vi "All stations power supply ID config.vi"(10 "station idx":i32, 11 "configuration file path":path) -> (0 "error out":errorcluster caption="错误输出", 2 "station idx":i32, 3 "configuration file path":path, 5 "one state power supply":T1={"VISA name CH"="", "Voltage Level (12 V)"=14.0, "Current Level (30 A)"=30.0})   [LabVIEW 2018]
uses:
  Crl defs/one state power supply config.ctl
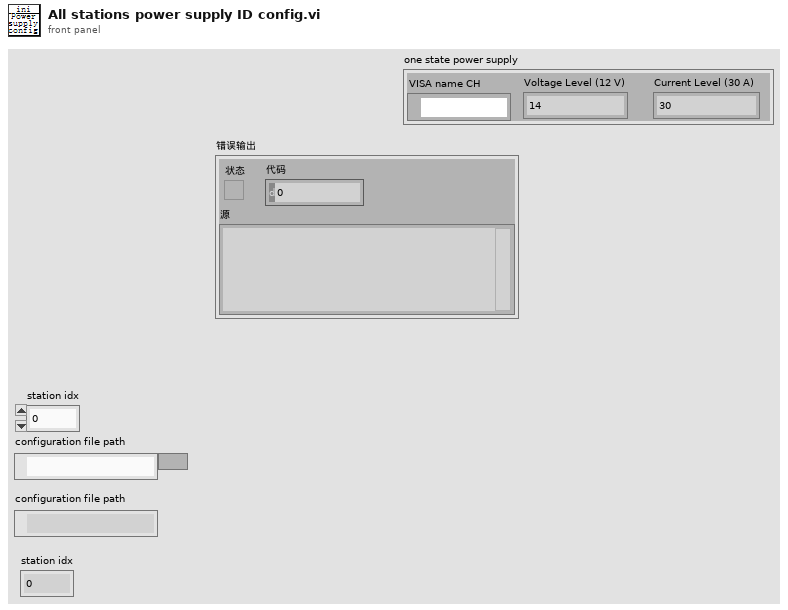
[diagram p1: front panel]
types:
  T1 = typedef "one state power supply config.ctl" = cluster{"VISA name CH":refnum<visa-resource-name>, "Voltage Level (12 V)":dbl, "Current Level (30 A)":dbl}
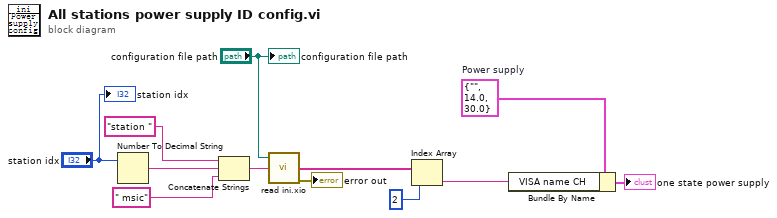
[diagram p0: block diagram]
diagram:
  w3 = T1 {"VISA name CH"="", "Voltage Level (12 V)"=14.0, "Current Level (30 A)"=30.0}  # Power supply
  n1 = Number To Decimal String(number="station idx") -> (decimal integer string=w10:string)  [unwired: 1 in]
  n2 = Concatenate Strings("station ", w10, " msic" ("string")) -> (w7:string)
  n3 = call "read ini.xio.vi"("configuration file path"="configuration file path", "Sections"=w7) -> ("Values"=w8:string[], "error out"=→"error out":errorcluster)  [unwired: 1 in, 3 out]
  n4 = Index Array(array=w8, index=2 ("索引")) -> (element=w2:string)
  n5 = Bundle By Name(cluster=w3, "VISA name CH"=w2) -> (→"one state power supply":T1)
  "configuration file path" <- "configuration file path"
  "station idx" <- "station idx"
